vi "Configure File Size Limit.vi"(8 "Error In":errorcluster, 11 "File Size Limit (Bytes)":i32) -> (0 "Error Out":errorcluster)   [LabVIEW 2014, in "Logger.lvlib"]
uses:
  Logger.lvlib
  Private/File/_Action.ctl
  Private/File/File.lvlib
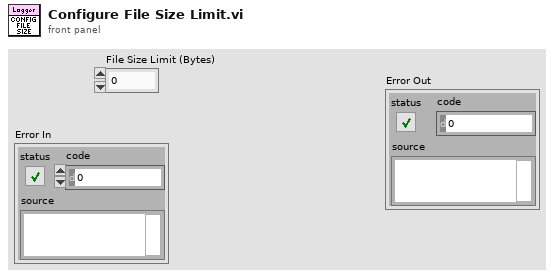
[diagram p1: front panel]
types:
  T1 = typedef "Logger.lvlib/File.lvlib/_Action.ctl" = enum16{"Initialize", "Set File Size Limit", "Set Root Folder", "Start", "Write", "Stop", "Shutdown"}
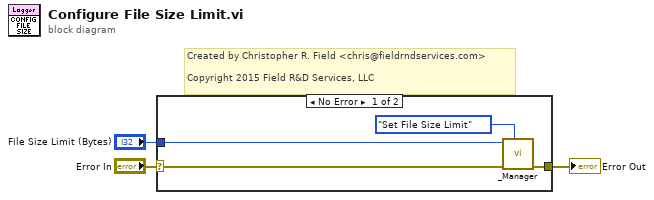
[diagram p0: block diagram]
diagram:
  # "Created by Christopher R. Field <chris@fieldrndservices.com>\n\nCopyright 2015 Field R&D Services, LLC"
  n1 = case shown="No Error" "Error In" {
    selector: "Error In" -> [w5 w8]
    tunnel: [w6 w8] -> w2
    tunnel: "File Size Limit (Bytes)" -> [w4 _]
    frame No Error {
      n2 = call "_Manager.vi"("Action"=_Action."Set File Size Limit", "Error In"=w5, "Set Value"=w4) -> ("Error Out"=w6:errorcluster)  [unwired: 8 in]
    }
    frame Error {
    }
  }
  "Error Out" <- w2
